vi "Filter Entity Paths OoC.vi"(11 "Class Paths":path[](array[path])) -> (1 "Classes":string[](array[string]), 2 "Names":string[](array[string]), 3 "Entity Paths":path[](array[path]))   [LabVIEW 2020, in "Conditum-Tools.lvlib" / "Entity Editor.lvclass"]
uses:
  Entity Editor.lvclass
  <vilib>/IlluminatedG/IG Conditum Base/Conditum/Entity/Entity.lvclass
  Entity Editor.lvclass/Entity Editor.ctl
panel:
  out "error out":errorcluster
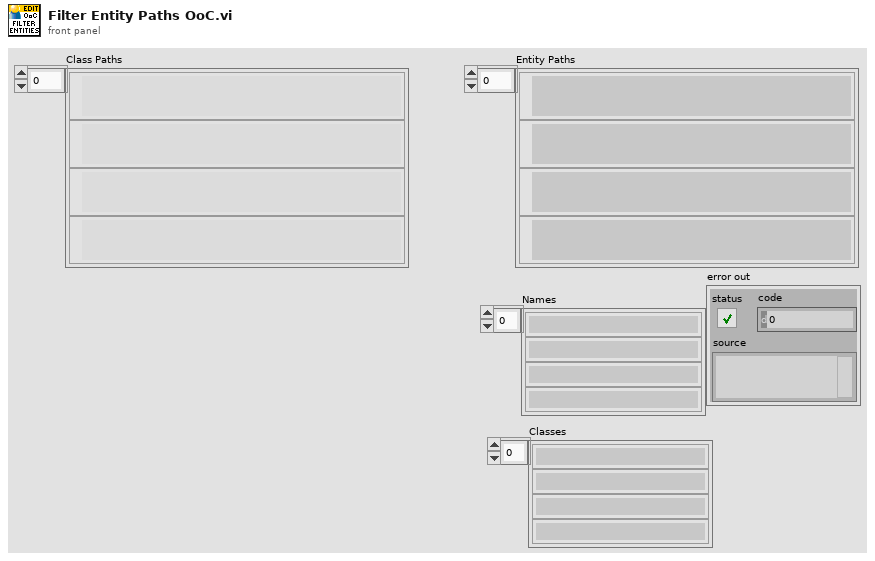
[diagram p1: front panel]
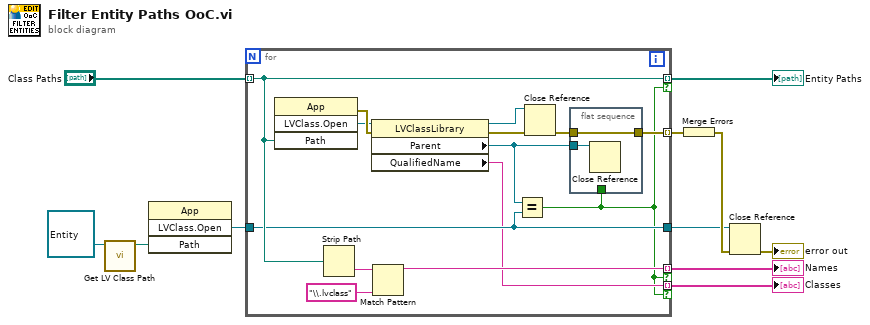
[diagram p0: block diagram]
diagram:
  n1 = call <vilib>:"Get LV Class Path.vi"("object"=refnum<class "Entity.lvclass"> refnum ("Conditum:Entity")) -> ("class path"=w8:path)  [unwired: 9 in, 1 out]
  n2 = invoke class="App" method="LVClass.Open"("Path"=w8) -> ("LVClass.Open"=w4:refnum<vi>)  [unwired: 3 in, 3 out]
  n3 = for {
    tunnel: "Class Paths" -> [w23] mode=indexing
    tunnel: w4 -> [w17]
    tunnel: [w23] -> w6 mode=indexing if=w12
    tunnel: [w20] -> w7 mode=indexing if=w12
    tunnel: [w15] -> w5 mode=indexing
    tunnel: [w17] -> w3
    tunnel: [w13] -> w1 mode=indexing if=w12
    n4 = invoke class="App" method="LVClass.Open"("Path"=w23) -> (error out=w25:errorcluster, "LVClass.Open"=w24:refnum<vi>)  [unwired: 3 in, 2 out]
    n5 = Strip Path(path=w23) -> (name=w22:string)  [unwired: 1 out]
    n6 = property class="LVClassLibrary"(reference=w24, error in=w25) -> (reference out=w18:refnum<vi>, error out=w19:errorcluster, "Parent"=w14:refnum<vi>, "QualifiedName"=w13:string)
    n7 = Match Pattern(string=w22, regular expression="\\.lvclass") -> (before substring=w20:string)  [unwired: 1 in, 3 out]
    n8 = Equal?(x=w14, y=w17) -> (x = y?=w12:bool)
    n9 = Close Reference(reference=w18, error in (no error)=w19) -> (error out=w16:errorcluster)
    n10 = flat-sequence {
      tunnel: w16 -> [w26]
      tunnel: [w26] -> w15
      tunnel: w14 -> [w27]
      tunnel: w12 -> [_]
      frame #0 {
        n11 = Close Reference(reference=w27) -> ()  [unwired: 1 in, 1 out]
      }
    }
  }
  "Entity Paths" <- w6
  "Names" <- w7
  "Classes" <- w1
  n12 = Merge Errors(w5) -> (w11:errorcluster)
  n13 = Close Reference(reference=w3, error in (no error)=w11) -> (error out=→"error out":errorcluster)
